vi "obj_ClientSrv Runlevels.vi"(0 "method":T1, 5 "LuaVIEW reference {initialize}":T2, 7 "runlevel":string, 11 "error in (no error)":errorcluster) -> (4 "names":string[](array[string]), 8 "current":string, 10 "script path":path, 15 "error out":errorcluster)   [LabVIEW 2012]
doc: "Holds and publishes some state for the runlevels module."
uses:
  typedefs/t_ClientSrv Runlevels Methods.ctl
  luaview/typedefs/t_LuaVIEW Reference.ctl
  luaview/subvis/private/LuaVIEW Pull (flat data).vi
  luaview/glb_LuaVIEW Configuration Globals.vi
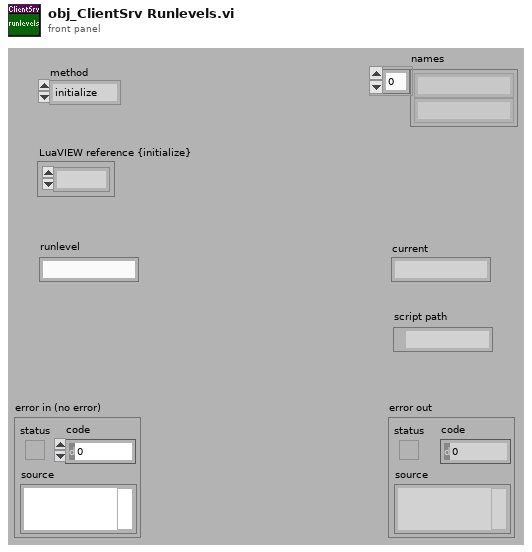
[diagram p1: front panel]
types:
  T1 = typedef "t_ClientSrv Runlevels Methods.ctl" = enum16{"initialize", "get path", "get levels", "get modes", "set current", "cleanup"}
  T2 = typedef "t_LuaVIEW Reference.ctl" = refnum<k1>
  T3 = cluster{"runlevel scripts":path[], "boot modes":string[]}
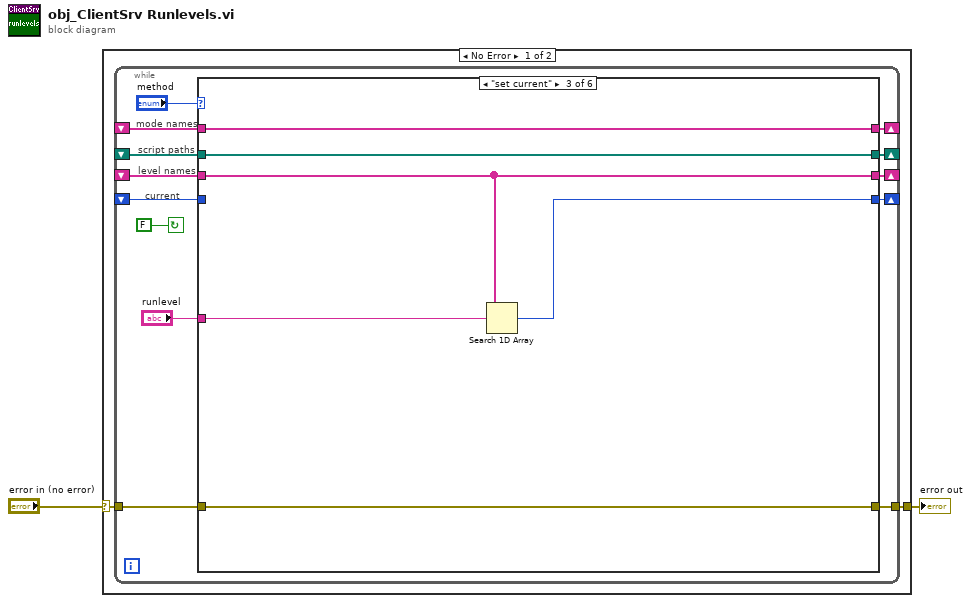
[diagram p0: block diagram]
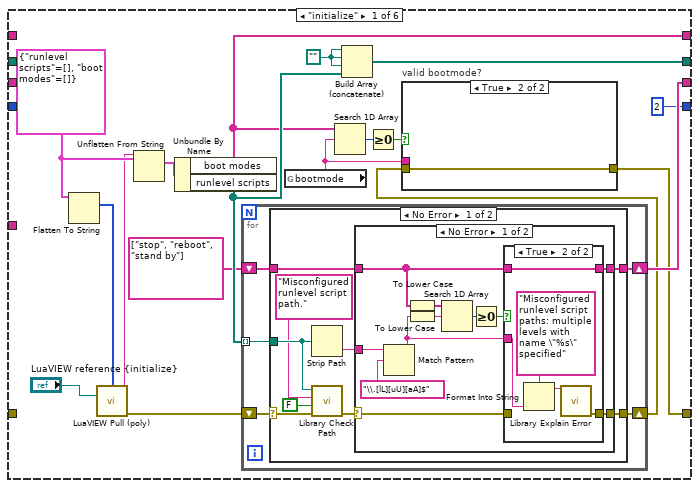
[diagram p2: hidden frame]
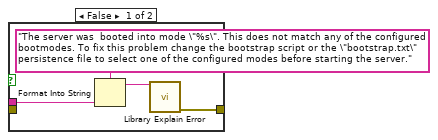
[diagram p3: hidden frame]
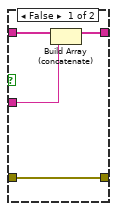
[diagram p4: hidden frame]
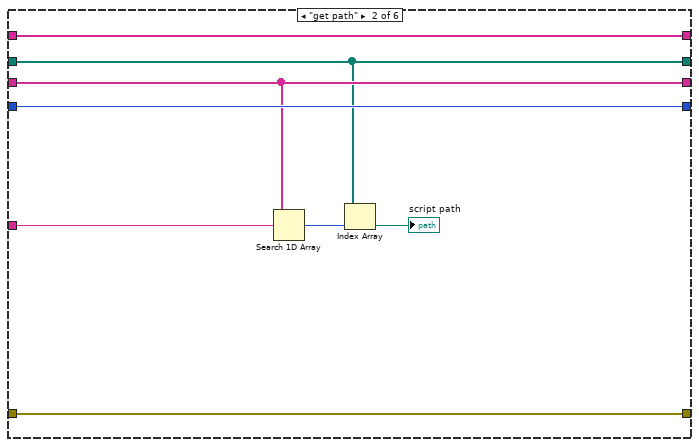
[diagram p7: hidden frame]
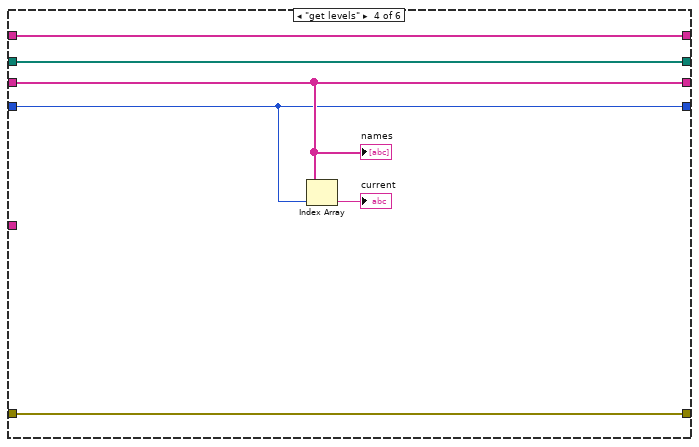
[diagram p8: hidden frame]
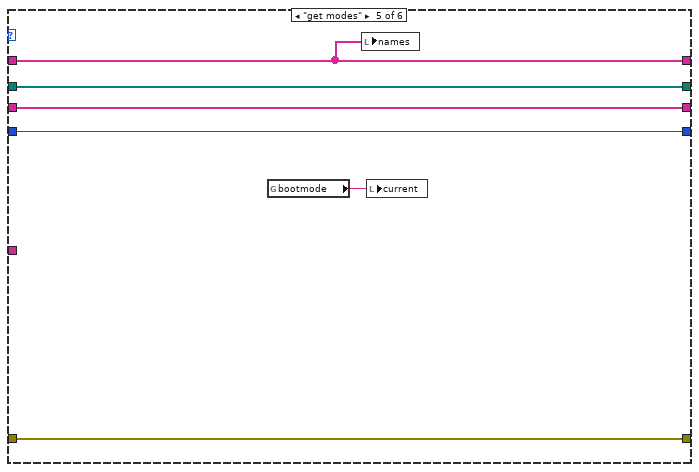
[diagram p9: hidden frame]
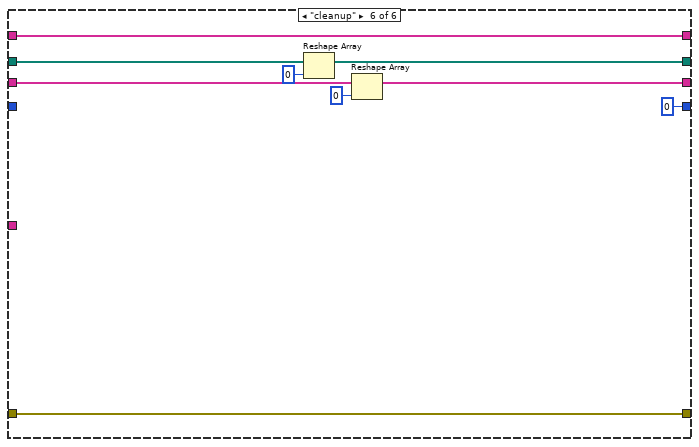
[diagram p10: hidden frame]
diagram:
  n1 = case shown="No Error" "error in (no error)" {
    selector: "error in (no error)" -> [w4 w114]
    tunnel: [w3 w114] -> w1
    frame No Error {
      n2 = while {
        tunnel: w4 -> [w17]
        tunnel: [w16] -> w3
        shift-right: [w14] -> _
        shift-left: _ -> [w15]
        shift-right: [w11] -> _
        shift-left: _ -> [w10]
        shift-right: [w9] -> _
        shift-left: _ -> [w8]
        shift-right: [w5] -> _
        shift-left: _ -> [w6]
        stop <- FALSE continue-if-true
        # "mode names"
        # "current"
        # "level names"
        # "script paths"
        n3 = case shown="\"set current\"" "method" {
          tunnel: w17 -> [_ w86 w92 w98 w104 w112]
          tunnel: [w18 w86 w92 w98 w104 w112] -> w16
          tunnel: w15 -> [_ w83 w90 w97 w103 w113]
          tunnel: [w26 w83 w90 w97 w103 w110] -> w14
          tunnel: [w29 w84 w91 w95 w102 w106] -> w11
          tunnel: w10 -> [_ w84 w91 w95 w102 w107]
          tunnel: [2 w85 w88 w94 w101 0] -> w9
          tunnel: w8 -> [_ w85 _ w94 w101 _]
          tunnel: "runlevel" -> [_ w80 w89 _ _ _]
          tunnel: w6 -> [_ w79 w87 w93 w100 w105]
          tunnel: [w24 w79 w87 w93 w100 w105] -> w5
          frame "initialize" {
            w25 = path ""
            w34 = T3 {"runlevel scripts"=[], "boot modes"=[]} ("server access config out")
            n4 = Flatten To String(anything=w34) -> (type string=w35:i16[])  [unwired: 3 in, 2 out]
            n5 = call-poly "LuaVIEW Pull (poly).vi"("type descriptor"=w35, "LuaVIEW reference in"="LuaVIEW reference {initialize}") -> ("flat data"=w33:string, "error out"=w20:errorcluster)  [unwired: 11 in, 1 out]
            n6 = Unflatten From String(type=w34, binary string=w33) -> (value=w31:T3)  [unwired: 3 in, 2 out]
            n7 = Unbundle By Name(w31) -> ("boot modes"=w24:string[], "runlevel scripts"=w30:path[])
            n8 = for {
              tunnel: w30 -> [w44] mode=indexing
              shift-right: [w45] -> w19
              shift-left: w20 -> [w43]
              shift-right: [w41] -> w29
              shift-left: string[] ["stop", "reboot", "stand by"] -> [w42]
              n9 = case shown="No Error" w43 {
                selector: w43 -> [w51 w78]
                tunnel: [w47 w78] -> w45
                tunnel: w44 -> [w53 _]
                tunnel: w42 -> [w49 w77]
                tunnel: [w48 w77] -> w41
                frame No Error {
                  n10 = Strip Path(path=w53) -> (name=w52:string)  [unwired: 1 out]
                  n11 = call "Library Check Path.vi"("error in (no error)"=w51, "directory (true)"=FALSE, "further explanation (none)"="Misconfigured runlevel script path.", "path"=w53) -> ("error out"=w50:errorcluster)  [unwired: 2 in, 1 out]
                  n12 = case shown="No Error" w50 {
                    selector: w50 -> [w55 w75]
                    tunnel: w52 -> [w64 _]
                    tunnel: w49 -> [w57 w76]
                    tunnel: [w60 w76] -> w48
                    tunnel: [w56 w75] -> w47
                    frame No Error {
                      n13 = Match Pattern(string=w64, regular expression="\\.[lL][uU][aA]$") -> (before substring=w59:string)  [unwired: 1 in, 3 out]
                      n14 = To Lower Case(string=w57) -> (all lower case string=w58:string[])
                      n15 = To Lower Case(string=w59) -> (all lower case string=w63:string)
                      n16 = Search 1D Array(1D array=w58, element=w63) -> (index of element=w62:i32)  [unwired: 1 in]
                      n17 = Greater Or Equal To 0?(x=w62) -> (x >= 0?=w61:bool)
                      n18 = case shown="True" w61 {
                        tunnel: w57 -> [w69 w74]
                        tunnel: [w67 w74] -> w60
                        tunnel: w59 -> [w68 w71]
                        tunnel: [w66 w73] -> w56
                        tunnel: w55 -> [w66 _]
                        frame False {
                          n19 = Build Array (concatenate)(w69, w68) -> (w67:string[])
                        }
                        frame True {
                          n20 = Format Into String(format string="Misconfigured runlevel script paths: multiple levels with name \"%s\" specified", w71) -> (resulting string=w72:string)  [unwired: 2 in, 1 out]
                          n21 = call "Library Explain Error.vi"("explanation prefix (none)"=w72) -> ("explained error"=w73:errorcluster)  [unwired: 14 in]
                        }
                      }
                    }
                    frame Error {
                    }
                  }
                }
                frame Error {
                }
              }
            }
            n22 = global read "glb_LuaVIEW Configuration Globals.vi" "bootmode"() -> (w21:string)
            n23 = Search 1D Array(1D array=w24, element=w21) -> (index of element=w23:i32)  [unwired: 1 in]
            n24 = Build Array (concatenate)(w25, w25, w25, w30) -> (w26:path[])
            n25 = Greater Or Equal To 0?(x=w23) -> (x >= 0?=w22:bool)
            n26 = case "valid bootmode?" shown="True" w22 {
              tunnel: w21 -> [w39 _]
              tunnel: w19 -> [_ w40]
              tunnel: [w38 w40] -> w18
              frame False {
                n27 = Format Into String(format string="The server was  booted into mode \"%s\". This does not match any of the configured bootmodes. To fix this problem change the bootstrap script or the \"bootstrap.txt\" persistence file to select one of the configured modes before starting the server.", w39) -> (resulting string=w37:string)  [unwired: 2 in, 1 out]
                n28 = call "Library Explain Error.vi"("explanation prefix (none)"=w37) -> ("explained error"=w38:errorcluster)  [unwired: 14 in]
              }
              frame True {
              }
            }
          }
          frame "get path" {
            n29 = Search 1D Array(1D array=w84, element=w80) -> (index of element=w82:i32)  [unwired: 1 in]
            n30 = Index Array(array=w83, index=w82) -> (element=→"script path":path)
          }
          frame "set current" {
            n31 = Search 1D Array(1D array=w91, element=w89) -> (index of element=w88:i32)  [unwired: 1 in]
          }
          frame "get levels" {
            n32 = Index Array(array=w95, index=w94) -> (element=→"current":string)
            "names" <- w95
          }
          frame "get modes" {
            n33 = global read "glb_LuaVIEW Configuration Globals.vi" "bootmode"() -> (w99:string)
            n34 = local write "names"(w100) -> ()
            n35 = local write "current"(w99) -> ()
          }
          frame "cleanup" {
            n36 = Reshape Array(w113, 0 ("dimension size")) -> (w110:path[])
            n37 = Reshape Array(w107, 0 ("dimension size")) -> (w106:string[])
          }
        }
      }
    }
    frame Error {
    }
  }
  "error out" <- w1
